vi "visa read.vi"(8 "error in":errorcluster, 9 "字节总数":u32, 10 "delay before read (ms)":u32=500, 11 "VISA resource name in":refnum<visa-resource-name>) -> (0 "error out":errorcluster, 1 "return count":dbl, 2 "String of array":string, 3 "VISA resource name out":refnum<visa-resource-name>)   [LabVIEW 2015, in "485 comm Custom Device.lvlib"]
doc: "This example performs a serial port write and a serial port read. The parameters set for the serial port must match the parameters of the connected instrument or device. The VISA Configure Serial Port VI sets the configuration parameters. The front panel displays the controls used to configure the basic parameters, such as baud rate, data bits, and parity. The VI passes the VISA resource name to other VIs that perform operations on that VISA resource. The VISA Write function sends a command to the serial device and the VISA Read function returns data based on the command. The VISA Close function then closes the reference to the serial device. It is important to close the reference; otherwise, further communication through that port might not be possible."
uses:
  485 comm Custom Device.lvlib
panel:
  out "bytes read":u32
  out "Response":string
  # "Overview: Demonstrates the use of the VISA functions to send a single command to a serial instrument and read a response.\nRequirements: NI-VISA Driver\nInstructions:\n1. Ensure the resource specified by the VISA resource name is a valid serial device.\n2. Run the VI.\n3. If your instrument recognizes the \"*IDN?\" command, it should return a Response."
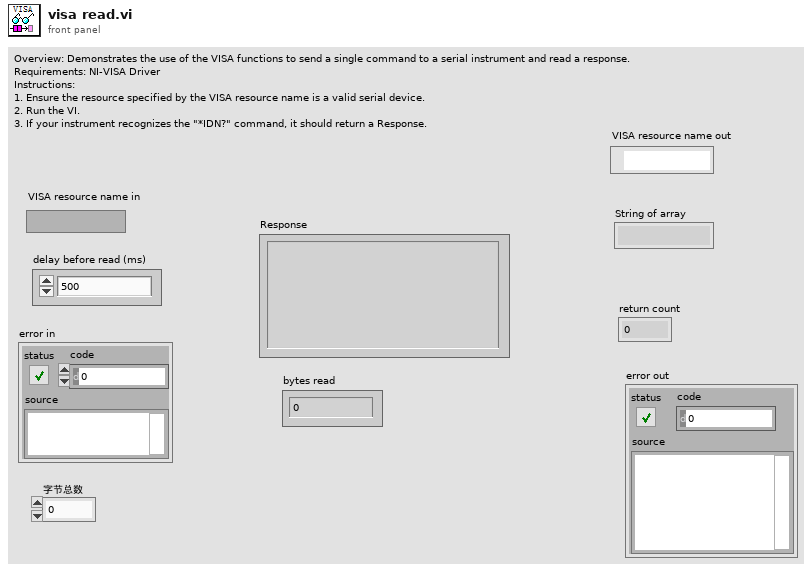
[diagram p1: front panel]
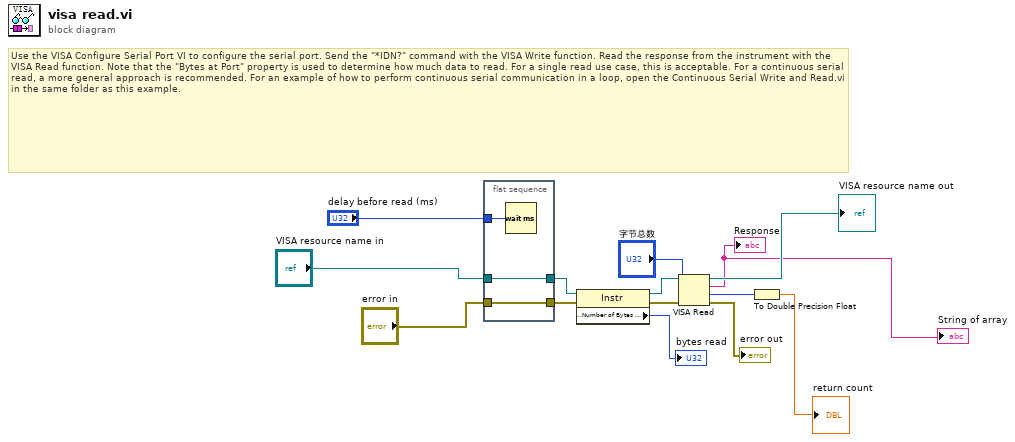
[diagram p0: block diagram]
diagram:
  # "Use the VISA Configure Serial Port VI to configure the serial port. Send the \"*IDN?\" command with the VISA Write function. Read the response from the instrument with the VISA Read function. Note that the \"Bytes at Port\" property is used to determine how much data to read. For a single read use case, this is acceptable. For a continuous serial read, a more general approach is recommended. For an example of how to perform continuous serial communication in a loop, open the Continuous Serial Write and Read.vi in the same folder as this example."
  n1 = flat-sequence {
    tunnel: "error in" -> [w16]
    tunnel: [w16] -> w14
    tunnel: "VISA resource name in" -> [w15]
    tunnel: [w15] -> w13
    tunnel: "delay before read (ms)" -> [w17]
    frame #0 {
      n2 = Wait (ms)(milliseconds to wait=w17) -> ()  [unwired: 1 out]
    }
  }
  n3 = property class="Instr"(reference=w13, error in=w14) -> (reference out=w11:refnum<visa-resource-name>, error out=w10:errorcluster, "Serial Settings:Number of Bytes at Serial Port"=→"bytes read":u32)
  n4 = VISA Read(VISA resource name=w11, byte count="字节总数", error in (no error)=w10) -> (VISA resource name out=→"VISA resource name out":refnum<visa-resource-name>, read buffer=→"Response" →"String of array":string, return count=w8:u32, error out=→"error out":errorcluster)
  n5 = To Double Precision Float(number=w8) -> (double precision float=→"return count":dbl)
